vi "P3Y2.vi"(2 "error in (no error)":errorcluster) -> (0 "appended array":cluster{i32, i32, dbl[]}[](array[cluster]), 1 "error out":errorcluster)   [LabVIEW 2020]
doc: "Võtab argumentidena cos ja sin sagedust ja amplituuti. Lisaks vaadatavte punktide arvu. Tagastatakse masiiv koos andmetega"
panel:
  in  "cos amp":dbl
  in  "sin amp":dbl
  in  "cos sagedus":dbl
  in  "sin sagedus":dbl
  in  "Puntkide arv":i32
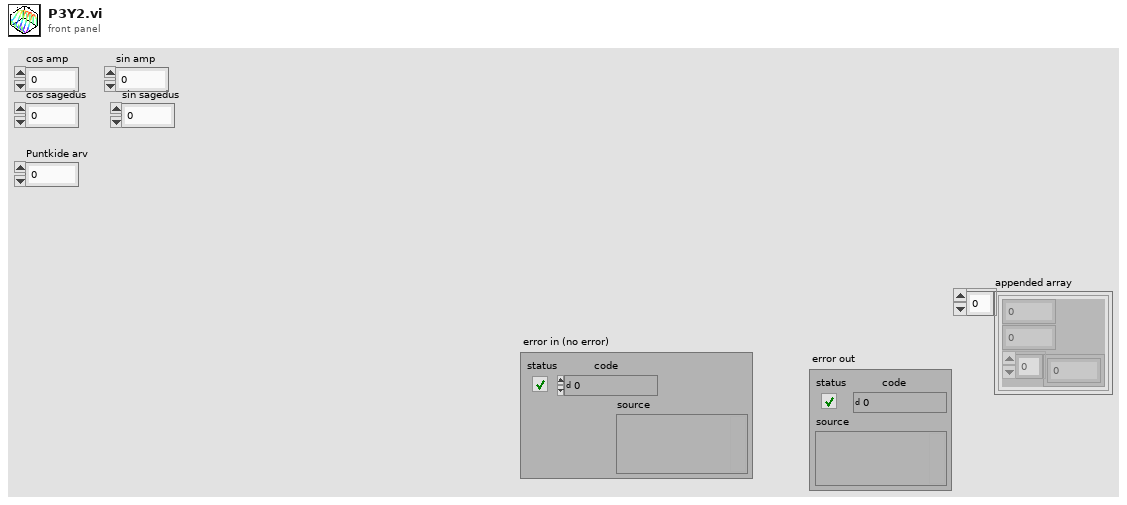
[diagram p1: front panel]
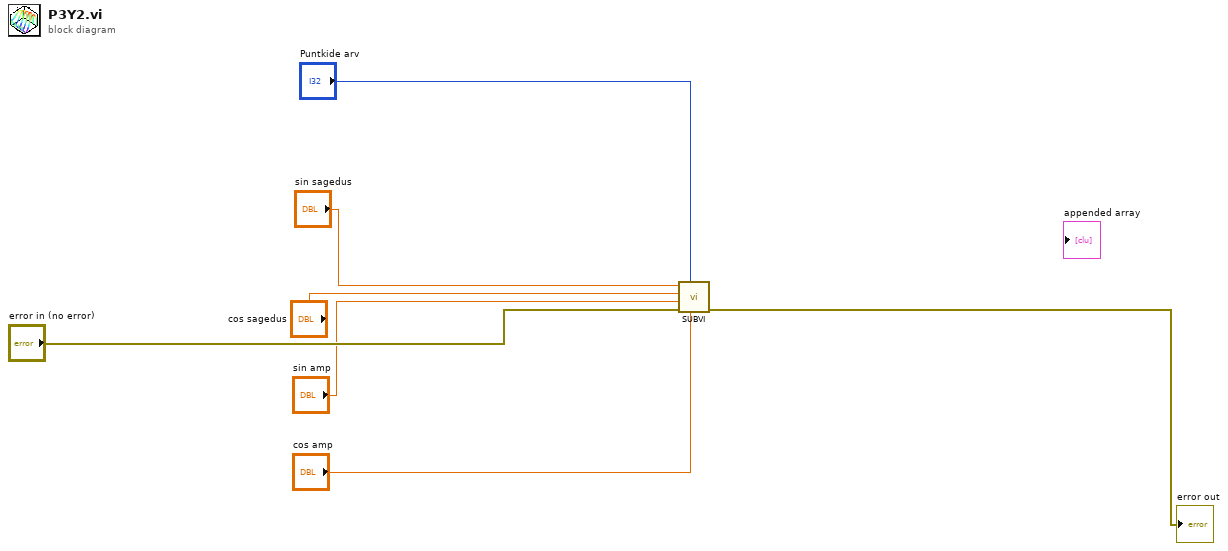
[diagram p0: block diagram]
diagram:
  n1 = call "SUBVI.vi"("cos amp"="cos amp", "Puntkide arv"="Puntkide arv", "error in (no error)"="error in (no error)", "sin amp"="sin amp", "cos sagedus"="cos sagedus", "sin sagedus"="sin sagedus") -> ("error out"=→"error out":errorcluster)  [unwired: 5 in]
